vi "DT_Cal Cos Angle.vi"(9 "p 3":cluster{"x":dbl, "y":dbl, "index":i32}, 10 "p 2":cluster{"x":dbl, "y":dbl, "index":i32}, 11 "p 1":cluster{"x":dbl, "y":dbl, "index":i32}) -> (3 "cos":dbl)   [LabVIEW 2020, in "NI_AAL_Geometry.lvlib"]
uses:
  <vilib>/Analysis/NI_AAL_Geometry.lvlib
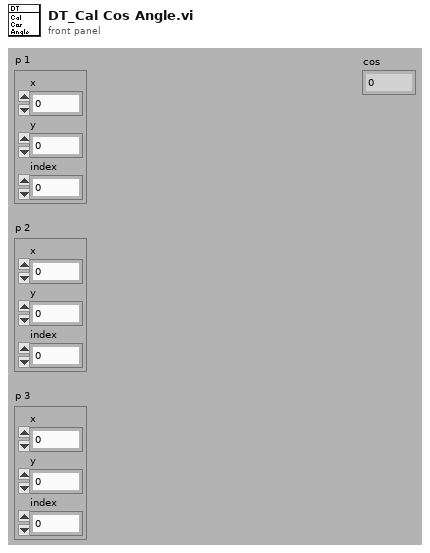
[diagram p1: front panel]
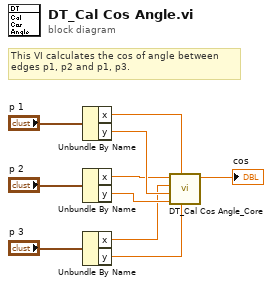
[diagram p0: block diagram]
diagram:
  # "This VI calculates the cos of angle between \nedges p1, p2 and p1, p3."
  n1 = Unbundle By Name("p 1") -> ("x"=w10:dbl, "y"=w9:dbl)
  n2 = Unbundle By Name("p 2") -> ("x"=w8:dbl, "y"=w7:dbl)
  n3 = Unbundle By Name("p 3") -> ("x"=w6:dbl, "y"=w5:dbl)
  n4 = call <vilib>:"DT_Cal Cos Angle_Core.vi"("y3"=w5, "x1"=w10, "y2"=w7, "y1"=w9, "x3"=w6, "x2"=w8) -> ("angle"=→"cos":dbl)  [unwired: 5 out]
